vi "kvCanGetDriverMode.vi"(0 "Channel Handle (input only)":i32, 1 "error in (no error)":errorcluster) -> (2 "Channel Handle (output only)":i32, 3 "Driver Mode":i32(ring) items=["Not Available", "Reserve 1", "Reserve 2", "Reserve 3", "SWC Sleep Mode", "SWC Normal Mode", "SWC High-Speed Mode", "SWC Wakeup Mode", "Sleep Mode", "Normal Mode", "Standby Mode", "Truck & Trailer: CAN High Mode", "Truck & Trailer: CAN Low Mode", "Reserved OEM 1", "Reserved OEM 2", "Reserved OEM 3", "Reserved OEM 4"], 4 "ResNet Mode":i32, 5 "error out":errorcluster)   [LabVIEW 2022 SP3]
doc: "This function retrieves the current CAN bus driver mode. This is typically a mode like sleep, wakeup, standby, fast mode, etc. The different modes are almost always hardware dependent and requires special DRVcan cables. As an example, the DRVcan S implements J2411 compliant single-wire CAN and supports four line modes, namely Normal, Sleep, Fast and Wakeup.\n\nStandard ISO 11898 CAN do not support any of these bus driver modes."
uses:
  canlib32.dll
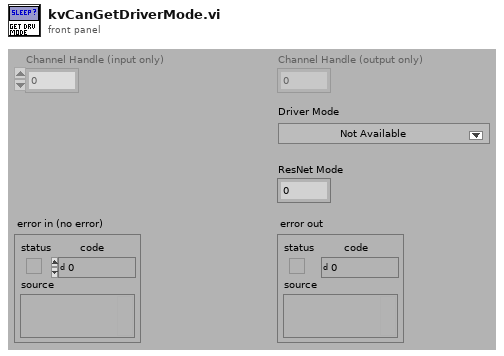
[diagram p1: front panel]
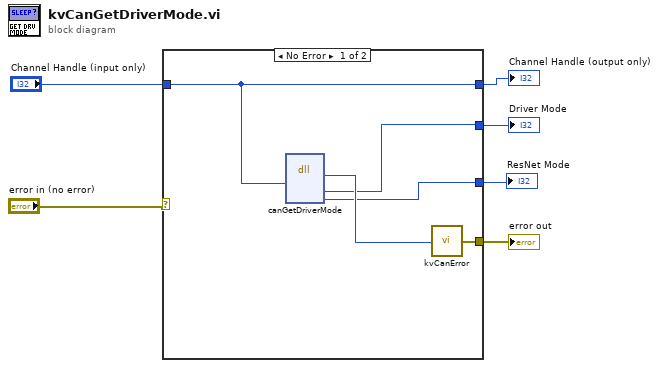
[diagram p0: block diagram]
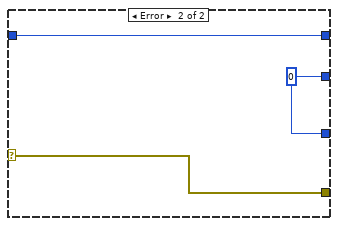
[diagram p2: hidden frame]
diagram:
  n1 = case shown="No Error" "error in (no error)" {
    selector: "error in (no error)" -> [_ w12]
    tunnel: "Channel Handle (input only)" -> [w7 w14]
    tunnel: [w7 w14] -> w4
    tunnel: [w9 w13] -> w3
    tunnel: [w8 w13] -> w2
    tunnel: [w11 w12] -> w1
    frame No Error {
      n2 = dll-call lib="canlib32.dll" fn="canGetDriverMode"("channelHandle"=w7) -> (w10:i32, "lineMode"=w9:i32, "resNet"=w8:i32)  [unwired: 6 in, 2 out]
      n3 = call "kvCanError.vi"("error code"=w10) -> ("error out"=w11:errorcluster)
    }
    frame Error {
      w13 = 0
    }
  }
  "Channel Handle (output only)" <- w4
  "error out" <- w1
  "Driver Mode" <- w3
  "ResNet Mode" <- w2
